vi "PS Control-alternate.vi"() -> ()   [LabVIEW 2020]
panel:
  out "Power Supply State":T1(ring)
  out "Output Cluster":T2 {"MaxLambdaCurrent [A]" format="%.2f"; "LambdaRates [A/min]" format="%.5e"; "MaxNormalCurrent [A]" format="%.2f"; "StabilitySetting [%]" format="%.2f"; "FieldCurrentRatio [T/A]" format="%.2f"; "SwitchWaitTime [s]" format="%.2f"; "SwitchHtrCurrent [mA]" format="%.2f"; "TrainRates [A/min]" format="%.5e"; "NormalRates [A/min]" format="%.5e"; "Breakpts [A]" format="%.5e"}
  in  "Local Enable":bool
  in  "Lambda Mode":bool
  in  "Training Mode":bool
  out "Lambda":bool
  out "Train":bool
  out "Persistent Field":dbl format="%.4f"
  out "Persistence Status":string
  out "Persistent":bool
  in  "Return from persistence":bool
  in  "Make Persistent":bool
  in  "Ramp to Zero":bool
  in  "Hold":bool
  in  "Ramp to Setpoint":bool
  in  "Rate [T/min]":dbl min=0.0 max=5.0 step=0.1 format="%.5f"
  in  "Setpoint [T]":dbl format="%.5f"
  out "Magnet \nVoltage":dbl format="%.2f"
  out "Field [T]":dbl format="%.4f"
  out "Switch Heater Error":bool
  out "Switch heater \nconfirmed":bool
  out "Switch Heater":bool
  in  "VISA session":refnum<visa-resource-name>="GPIB0::22::INSTR"
  in  "stop":bool
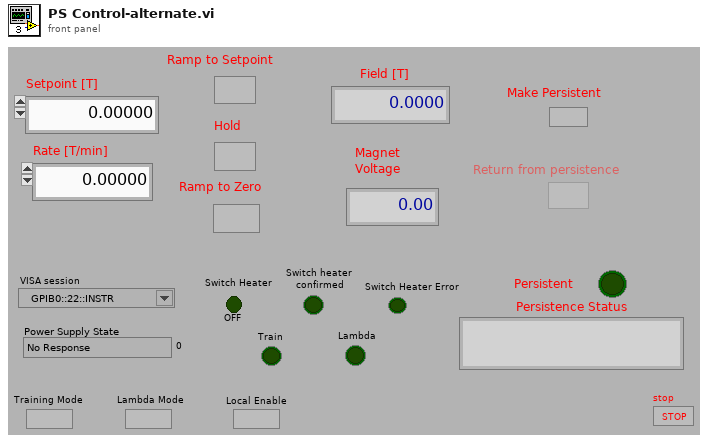
[diagram p1: front panel]
types:
  T1 = enum16{"No Response", "Ramping to programmed field ", "Holding at programmed field", "Paused", "Ramp Manual Up", "Ramp Manual Down", "Ramping to Zero", "QUENCH", "Heating Persistence Switch", "At Zero Current"}
  T2 = cluster{"Breakpts [A]":dbl[], "NormalRates [A/min]":dbl[], "TrainRates [A/min]":dbl[], "SwitchHtrCurrent [mA]":dbl, "SwitchWaitTime [s]":dbl, "FieldCurrentRatio [T/A]":dbl, "StabilitySetting [%]":dbl, "MaxNormalCurrent [A]":dbl, "Magnet ID":string, "LambdaRates [A/min]":dbl[], "MaxLambdaCurrent [A]":dbl}
  T3 = enum16{"Normal", "Train", "Lambda", "Train & Lambda"}
  T4 = enum8{"Enabled", "Disabled", "Disabled and Grayed Out"}
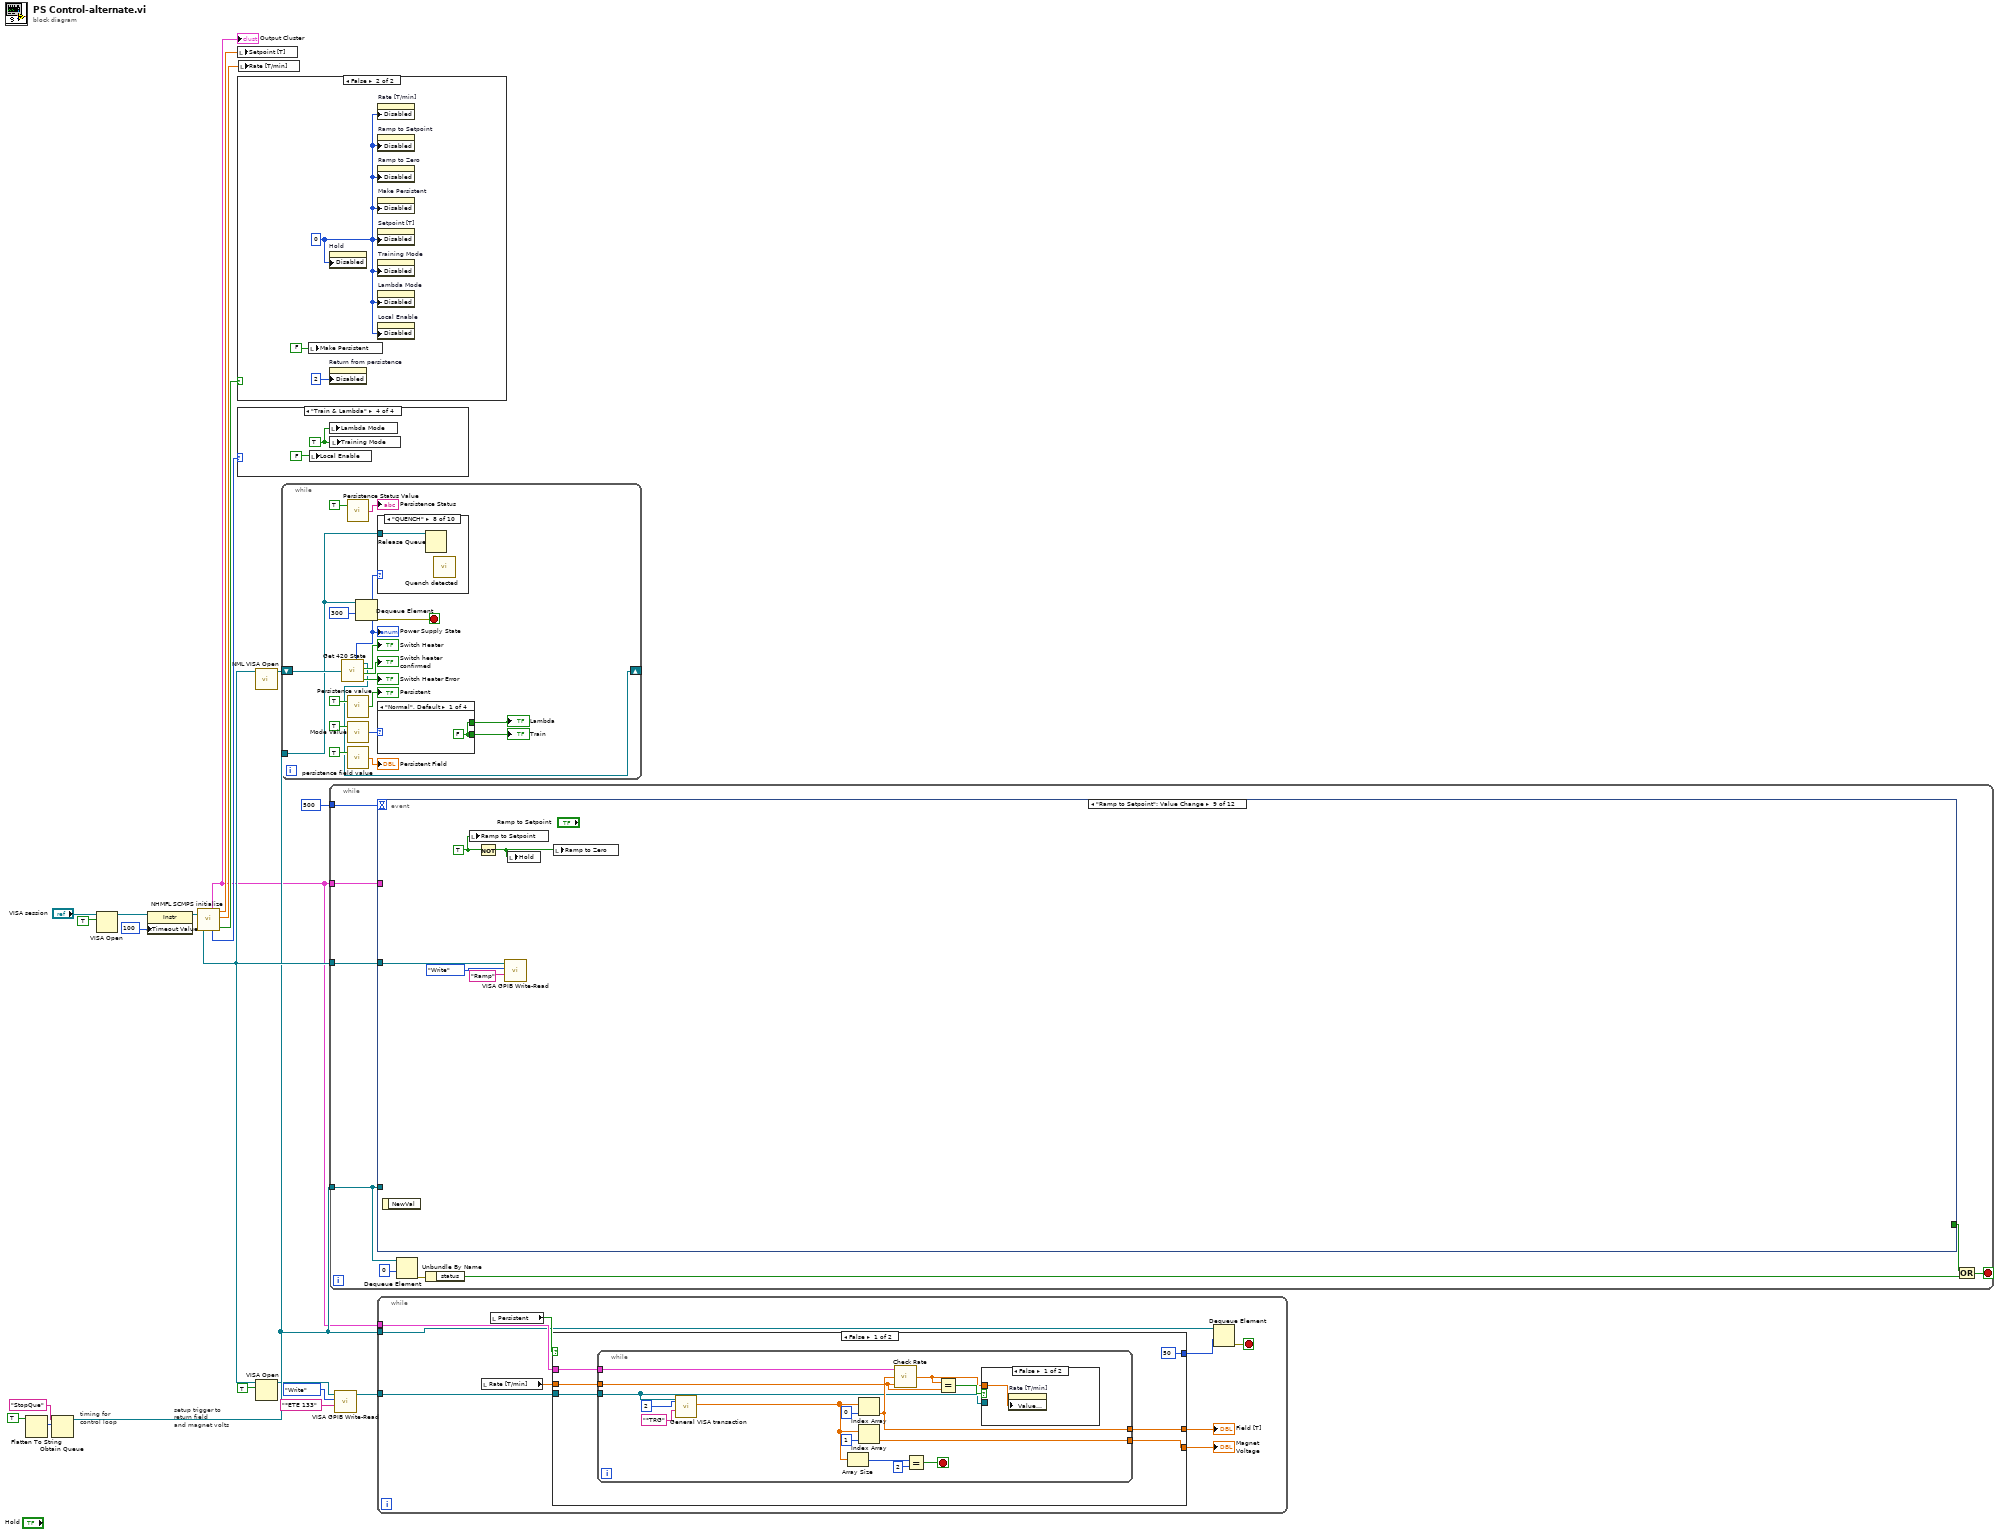
[diagram p0: block diagram]
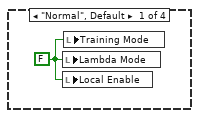
[diagram p2: hidden frame]
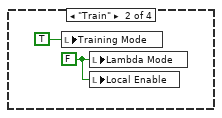
[diagram p3: hidden frame]
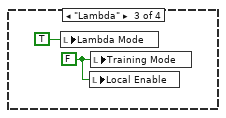
[diagram p4: hidden frame]
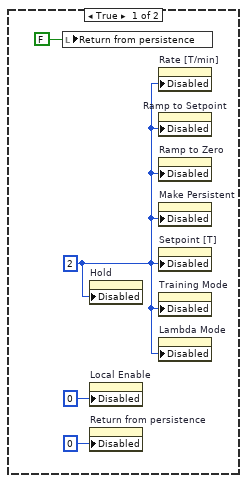
[diagram p5: hidden frame]
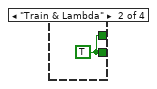
[diagram p15: hidden frame]
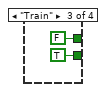
[diagram p16: hidden frame]
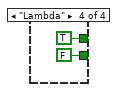
[diagram p17: hidden frame]
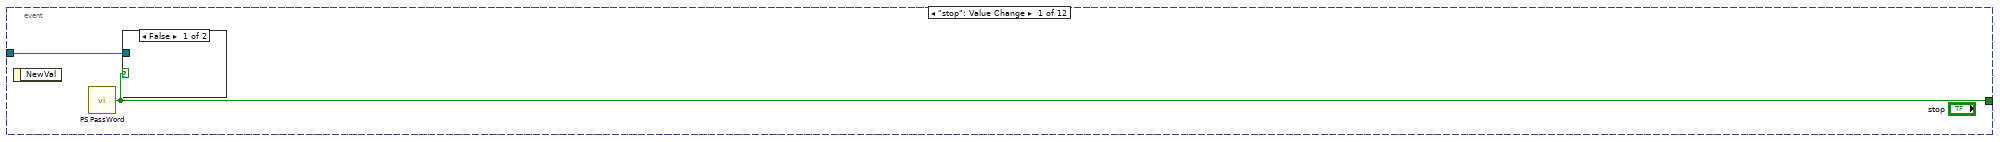
[diagram p18: hidden frame]
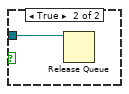
[diagram p19: hidden frame]
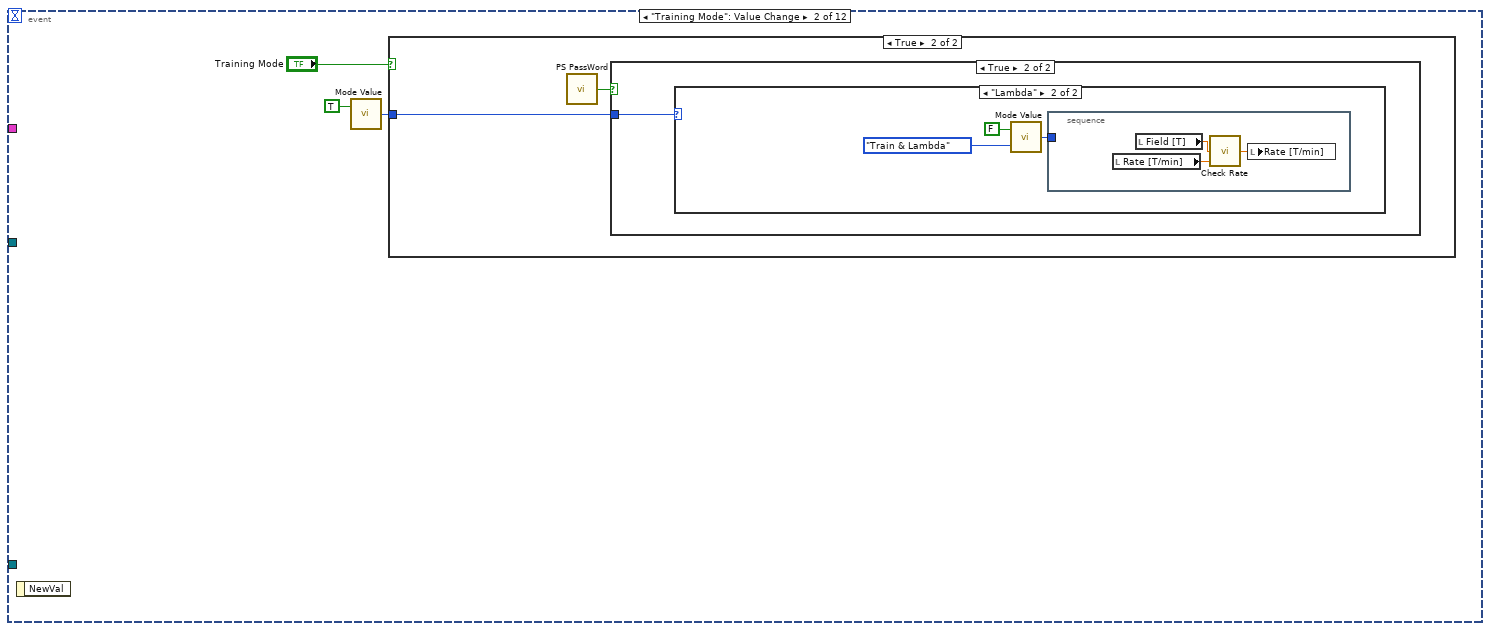
[diagram p20: hidden frame]
diagram:
  # "timing for \ncontrol loop"
  # "setup trigger to \nreturn field\nand magnet volts"
  n1 = Flatten To String(anything=TRUE) -> (type string=w18:i16[])  [unwired: 3 in, 2 out]
  n2 = Obtain Queue(name (unnamed)="StopQue", element data type=w18) -> (queue out=w13:refnum<queue>)  [unwired: 3 in, 2 out]
  n3 = VISA Open(duplicate session (F)=TRUE, VISA resource name="VISA session") -> (VISA resource name=w2:refnum<visa-resource-name>)  [unwired: 3 in, 1 out]
  n4 = property class="Instr"(reference=w2, "General Settings:Timeout Value"=u32 100) -> (reference out=w6:refnum<visa-resource-name>)  [unwired: 1 in, 1 out]
  n5 = call "NHMFL SCMPS initialize.vi"("VISA session"=w6) -> ("dup VISA session"=w14:refnum<visa-resource-name>, "Output Cluster"=w9:T2, "Mode Out"=w11:T3, "Programmed Field"=w16:dbl, "Ramp Rate"=w10:dbl, "Persistent"=w12:bool)  [unwired: 1 out]
  "Output Cluster" <- w9
  n6 = local write "Setpoint [T]"(w16) -> ()
  n7 = case shown="False" w12 {
    frame True {
      w24 = 2
      n8 = local write "Return from persistence"(FALSE ("Return from persistence")) -> ()
      n9 = property on="Hold" class="Bool (strict)"("Disabled"=w24) -> ()  [unwired: 2 in, 2 out]
      n10 = property on="Local Enable" class="Bool (strict)"("Disabled"=u8 0) -> ()  [unwired: 2 in, 2 out]
      n11 = property on="Return from persistence" class="Bool (strict)"("Disabled"=u8 0) -> ()  [unwired: 2 in, 2 out]
      n12 = property on="Rate [T/min]" class="DigNum (strict)"("Disabled"=w24) -> ()  [unwired: 2 in, 2 out]
      n13 = property on="Ramp to Setpoint" class="Bool (strict)"("Disabled"=w24) -> ()  [unwired: 2 in, 2 out]
      n14 = property on="Ramp to Zero" class="Bool (strict)"("Disabled"=w24) -> ()  [unwired: 2 in, 2 out]
      n15 = property on="Make Persistent" class="Bool (strict)"("Disabled"=w24) -> ()  [unwired: 2 in, 2 out]
      n16 = property on="Setpoint [T]" class="DigNum (strict)"("Disabled"=w24) -> ()  [unwired: 2 in, 2 out]
      n17 = property on="Training Mode" class="Bool (strict)"("Disabled"=w24) -> ()  [unwired: 2 in, 2 out]
      n18 = property on="Lambda Mode" class="Bool (strict)"("Disabled"=w24) -> ()  [unwired: 2 in, 2 out]
    }
    frame False {
      w27 = 0
      n19 = local write "Make Persistent"(FALSE ("Return from persistence")) -> ()
      n20 = property on="Hold" class="Bool (strict)"("Disabled"=w27) -> ()  [unwired: 2 in, 2 out]
      n21 = property on="Return from persistence" class="Bool (strict)"("Disabled"=u8 2) -> ()  [unwired: 2 in, 2 out]
      n22 = property on="Rate [T/min]" class="DigNum (strict)"("Disabled"=w27) -> ()  [unwired: 2 in, 2 out]
      n23 = property on="Ramp to Setpoint" class="Bool (strict)"("Disabled"=w27) -> ()  [unwired: 2 in, 2 out]
      n24 = property on="Ramp to Zero" class="Bool (strict)"("Disabled"=w27) -> ()  [unwired: 2 in, 2 out]
      n25 = property on="Make Persistent" class="Bool (strict)"("Disabled"=w27) -> ()  [unwired: 2 in, 2 out]
      n26 = property on="Setpoint [T]" class="DigNum (strict)"("Disabled"=w27) -> ()  [unwired: 2 in, 2 out]
      n27 = property on="Training Mode" class="Bool (strict)"("Disabled"=w27) -> ()  [unwired: 2 in, 2 out]
      n28 = property on="Lambda Mode" class="Bool (strict)"("Disabled"=w27) -> ()  [unwired: 2 in, 2 out]
      n29 = property on="Local Enable" class="Bool (strict)"("Disabled"=w27) -> ()  [unwired: 2 in, 2 out]
    }
  }
  n30 = case shown="\"Train & Lambda\"" w11 {
    frame "Normal", Default {
      w30 = FALSE ("Training Mode")
      n31 = local write "Lambda Mode"(w30) -> ()
      n32 = local write "Local Enable"(w30) -> ()
      n33 = local write "Training Mode"(w30) -> ()
    }
    frame "Train" {
      w32 = FALSE
      n34 = local write "Training Mode"(TRUE) -> ()
      n35 = local write "Lambda Mode"(w32) -> ()
      n36 = local write "Local Enable"(w32) -> ()
    }
    frame "Lambda" {
      w33 = FALSE
      n37 = local write "Lambda Mode"(TRUE) -> ()
      n38 = local write "Local Enable"(w33) -> ()
      n39 = local write "Training Mode"(w33) -> ()
    }
    frame "Train & Lambda" {
      w35 = TRUE
      n40 = local write "Local Enable"(FALSE) -> ()
      n41 = local write "Lambda Mode"(w35) -> ()
      n42 = local write "Training Mode"(w35) -> ()
    }
  }
  n43 = local write "Rate [T/min]"(w10) -> ()
  n44 = call "NML VISA Open.vi"("VISA resource name"=w14) -> ("VISA resource name out"=w3:refnum<visa-resource-name>)  [unwired: 9 in, 1 out]
  n45 = VISA Open(duplicate session (F)=TRUE, VISA resource name=w14) -> (VISA resource name=w5:refnum<visa-resource-name>)  [unwired: 3 in, 1 out]
  n46 = while {
    tunnel: w13 -> [w41]
    shift-right: [w37] -> _
    shift-left: w3 -> [w53]
    stop <- w52 stop-if-true
    n47 = call "Get 420 State.vi"("VISA session"=w53) -> ("State"=w40:T1, "dup VISA session"=w37:refnum<visa-resource-name>, "Switch Heater"=→"Switch Heater":bool, "Switch heater \nconfirmed"=→"Switch heater \nconfirmed":bool, "Switch Heater Error"=→"Switch Heater Error":bool)  [unwired: 1 out]
    "Power Supply State" <- w40
    n48 = call "Persistence Status Value.vi"("Read/Write this vi"=TRUE) -> ("Persistence Status Out"=→"Persistence Status":string)  [unwired: 1 in]
    n49 = call "Persistence value.vi"("Read/Write this vi"=TRUE) -> ("Persistence Out"=→"Persistent":bool)  [unwired: 1 in]
    n50 = call "Mode Value.vi"("Read/Write this vi"=TRUE) -> ("Mode Out"=w45:T3)  [unwired: 1 in]
    n51 = call "persistence field value.vi"("Read/Write this vi"=TRUE) -> ("Persistent Field Out"=→"Persistent Field":dbl)  [unwired: 1 in]
    n52 = Dequeue Element(queue=w41, timeout in ms (-1)=300) -> (error out=w52:errorcluster)  [unwired: 1 in, 3 out]
    n53 = case shown="\"QUENCH\"" w40 {
      tunnel: w41 -> [_ _ _ _ _ _ _ w56 _ _]
      frame "No Response", Default {
      }
      frame "Ramping to programmed field " {
      }
      frame "Holding at programmed field" {
      }
      frame "Paused" {
      }
      frame "Ramp Manual Up" {
      }
      frame "Ramp Manual Down" {
      }
      frame "Ramping to Zero" {
      }
      frame "QUENCH" {
        n54 = Release Queue(queue=w56) -> ()  [unwired: 2 in, 3 out]
        n55 = call "Quench detected.vi"() -> ()  [unwired: 1 out]
      }
      frame "Heating Persistence Switch" {
      }
      frame "At Zero Current" {
      }
    }
    n56 = case shown="\"Normal\", Default" w45 {
      tunnel: [w57 w58 TRUE FALSE] -> w44
      tunnel: [w57 w58 FALSE TRUE] -> w43
      frame "Normal", Default {
        w57 = FALSE
      }
      frame "Train & Lambda" {
        w58 = TRUE
      }
      frame "Train" {
      }
      frame "Lambda" {
      }
    }
    "Train" <- w44
    "Lambda" <- w43
  }
  n57 = while {
    tunnel: w14 -> [w71]
    tunnel: 500 ("y") -> [w70]
    tunnel: w13 -> [w67]
    tunnel: w9 -> [w68]
    stop <- w65 stop-if-true
    n58 = event shown="[8] \"Ramp to Setpoint\": Value Change" {
      selector: _ -> [_ _ _ _ _ _ _ _ _ _ _ _]
      dyn-events: _ -> [_ _ _ _ _ _ _ _ _ _ _ _]
      timeout: w70 -> [_ _ _ _ _ _ _ _ _ _ _ _]
      tunnel: w71 -> [_ _ _ w125 w147 w190 w200 w224 w230 w233 w238 _]
      tunnel: w67 -> [w73 _ _ _ _ _ _ _ _ _ _ _]
      tunnel: [w72 _ _ _ _ _ _ _ _ _ _ _] -> w69
      tunnel: w68 -> [_ _ _ w124 w141 _ _ w221 _ _ _ _]
      event "stop": Value Change {
        n59 = event-data() -> ()  [unwired: 1 in, 1 out]
        n60 = call "PS PassWord.vi"() -> ("Password Correct"=w72:bool)  [unwired: 2 in]
        n61 = case shown="False" w72 {
          tunnel: w73 -> [_ w74]
          frame False {
          }
          frame True {
            n62 = Release Queue(queue=w74) -> ()  [unwired: 2 in, 3 out]
          }
        }
      }
      event "Training Mode": Value Change {
        n63 = event-data() -> ()  [unwired: 1 in, 1 out]
        n64 = call "Mode Value.vi"("Read/Write this vi"=TRUE) -> ("Mode Out"=w75:T3)  [unwired: 1 in]
        n65 = case shown="True" "Training Mode" {
          tunnel: w75 -> [w78 w83]
          frame False {
            n66 = case shown="\"Train\", Default" w78 {
              frame "Train", Default {
                n67 = call "Mode Value.vi"("Mode In"=T3."Normal", "Read/Write this vi"=FALSE) -> ()  [unwired: 1 out]
              }
              frame "Train & Lambda" {
                n68 = call "Mode Value.vi"("Mode In"=T3."Lambda", "Read/Write this vi"=FALSE) -> ()  [unwired: 1 out]
              }
            }
          }
          frame True {
            n69 = call "PS PassWord.vi"() -> ("Password Correct"=w84:bool)  [unwired: 2 in]
            n70 = case shown="True" w84 {
              tunnel: w83 -> [_ w86]
              frame False {
                n71 = local write "Training Mode"(FALSE ("Train")) -> ()
              }
              frame True {
                n72 = case shown="\"Lambda\"" w86 {
                  frame "Normal", Default {
                    n73 = call "Mode Value.vi"("Mode In"=T3."Train", "Read/Write this vi"=FALSE) -> ("Mode Out"=w87:T3)
                    n74 = stacked-sequence {
                      tunnel: w87 -> [_]
                      frame #0 {
                        n75 = local read "Rate [T/min]"() -> (w92:dbl)
                        n76 = local read "Field [T]"() -> (w91:dbl)
                        n77 = call "Check Rate.vi"("Rate"=w92, "Field"=w91) -> ("Checked Rate"=w90:dbl)  [unwired: 1 in]
                        n78 = local write "Rate [T/min]"(w90) -> ()
                      }
                    }
                  }
                  frame "Lambda" {
                    n79 = call "Mode Value.vi"("Mode In"=T3."Train & Lambda", "Read/Write this vi"=FALSE) -> ("Mode Out"=w93:T3)
                    n80 = stacked-sequence {
                      tunnel: w93 -> [_]
                      frame #0 {
                        n81 = local read "Rate [T/min]"() -> (w98:dbl)
                        n82 = local read "Field [T]"() -> (w97:dbl)
                        n83 = call "Check Rate.vi"("Rate"=w98, "Field"=w97) -> ("Checked Rate"=w96:dbl)  [unwired: 1 in]
                        n84 = local write "Rate [T/min]"(w96) -> ()
                      }
                    }
                  }
                }
              }
            }
          }
        }
      }
      event "Lambda Mode": Value Change {
        n85 = event-data() -> ()  [unwired: 1 in, 1 out]
        n86 = call "Mode Value.vi"("Read/Write this vi"=TRUE) -> ("Mode Out"=w99:T3)  [unwired: 1 in]
        n87 = case shown="False" "Lambda Mode" {
          tunnel: w99 -> [w102 w107]
          frame False {
            n88 = case shown="\"Lambda\", Default" w102 {
              frame "Lambda", Default {
                n89 = call "Mode Value.vi"("Mode In"=T3."Normal", "Read/Write this vi"=FALSE) -> ()  [unwired: 1 out]
              }
              frame "Train & Lambda" {
                n90 = call "Mode Value.vi"("Mode In"=T3."Train", "Read/Write this vi"=FALSE) -> ()  [unwired: 1 out]
              }
            }
          }
          frame True {
            n91 = call "PS PassWord.vi"() -> ("Password Correct"=w108:bool)  [unwired: 2 in]
            n92 = case shown="True" w108 {
              tunnel: w107 -> [_ w110]
              frame False {
                n93 = local write "Lambda Mode"(FALSE) -> ()
              }
              frame True {
                n94 = case shown="\"Train\"" w110 {
                  frame "Train" {
                    n95 = call "Mode Value.vi"("Mode In"=T3."Train & Lambda", "Read/Write this vi"=FALSE) -> ("Mode Out"=w111:T3)
                    n96 = stacked-sequence {
                      tunnel: w111 -> [_]
                      frame #0 {
                        n97 = local read "Rate [T/min]"() -> (w116:dbl)
                        n98 = local read "Field [T]"() -> (w115:dbl)
                        n99 = call "Check Rate.vi"("Rate"=w116, "Field"=w115) -> ("Checked Rate"=w114:dbl)  [unwired: 1 in]
                        n100 = local write "Rate [T/min]"(w114) -> ()
                      }
                    }
                  }
                  frame "Normal", Default {
                    n101 = call "Mode Value.vi"("Mode In"=T3."Lambda", "Read/Write this vi"=FALSE) -> ("Mode Out"=w117:T3)
                    n102 = stacked-sequence {
                      tunnel: w117 -> [_]
                      frame #0 {
                        n103 = local read "Rate [T/min]"() -> (w122:dbl)
                        n104 = local read "Field [T]"() -> (w121:dbl)
                        n105 = call "Check Rate.vi"("Rate"=w122, "Field"=w121) -> ("Checked Rate"=w120:dbl)  [unwired: 1 in]
                        n106 = local write "Rate [T/min]"(w120) -> ()
                      }
                    }
                  }
                }
              }
            }
          }
        }
      }
      event "Local Enable": Value Change {
        n107 = event-data() -> ("NewVal"=w123:bool)  [unwired: 1 in]
        n108 = case shown="False" w123 {
          tunnel: w125 -> [w127 w133]
          tunnel: w124 -> [_ w132]
          frame False {
            n109 = call "VISA GPIB Write-Read.vi"("Command"="SYST:REM" ("Command String"), "Action"=enum16{"Write", "Read", "Write & Read"}."Write", "VISA resource name"=w127) -> ("dup VISA Session"=w126:refnum<visa-resource-name>)  [unwired: 5 in, 3 out]
            n110 = stacked-sequence {
              tunnel: w126 -> [_]
              frame #0 {
                n111 = local write "Local Enable"(FALSE ("Local Enable")) -> ()
              }
            }
          }
          frame True {
            n112 = call "PS PassWord.vi"() -> ("Password Correct"=w131:bool)  [unwired: 2 in]
            n113 = case shown="True" w131 {
              tunnel: w133 -> [_ w136]
              tunnel: w132 -> [_ _]
              frame False {
                n114 = local write "Local Enable"(FALSE) -> ()
              }
              frame True {
                n115 = call "VISA GPIB Write-Read.vi"("Command"="SYST:LOC" ("Command String"), "Action"=enum16{"Write", "Read", "Write & Read"}."Write", "VISA resource name"=w136) -> ("dup VISA Session"=w135:refnum<visa-resource-name>)  [unwired: 5 in, 3 out]
                n116 = stacked-sequence {
                  tunnel: w135 -> [_]
                  frame #0 {
                    n117 = local write "Local Enable"(TRUE) -> ()
                  }
                }
              }
            }
          }
        }
      }
      event "Setpoint [T]": Value Change {
        n118 = event-data() -> ()  [unwired: 1 in, 1 out]
        n119 = call "Mode Value.vi"("Read/Write this vi"=TRUE) -> ("Mode Out"=w143:T3)  [unwired: 1 in]
        n120 = case shown="\"Train & Lambda\"" w143 {
          tunnel: "Setpoint [T]" -> [w151 w160 w170 w180]
          tunnel: w141 -> [w158 w168 w178 w188]
          tunnel: [w150 w162 w172 w182] -> w140
          frame "Normal", Default {
            n121 = Unbundle By Name(w158) -> ("MaxNormalCurrent [A]"=w156:dbl, "FieldCurrentRatio [T/A]"=w155:dbl)
            n122 = Multiply(x=w156, y=w155) -> (x*y=w157:dbl)
            n123 = Absolute Value(x=w151) -> (abs(x)=w154:dbl)
            n124 = In Range and Coerce(upper limit=w157, x=w154, lower limit=0.0) -> (coerced(x)=w152:dbl)  [unwired: 1 out]
            n125 = Sign(1:w151) -> (0:w149:dbl)
            n126 = Multiply(x=w152, y=w149) -> (x*y=w150:dbl)
          }
          frame "Train" {
            n127 = Unbundle By Name(w168) -> ("MaxNormalCurrent [A]"=w166:dbl, "FieldCurrentRatio [T/A]"=w165:dbl)
            n128 = Multiply(x=w166, y=w165) -> (x*y=w167:dbl)
            n129 = Absolute Value(x=w160) -> (abs(x)=w164:dbl)
            n130 = In Range and Coerce(upper limit=w167, x=w164, lower limit=0.0) -> (coerced(x)=w161:dbl)  [unwired: 1 out]
            n131 = Sign(1:w160) -> (0:w159:dbl)
            n132 = Multiply(x=w161, y=w159) -> (x*y=w162:dbl)
          }
          frame "Lambda" {
            n133 = Unbundle By Name(w178) -> ("MaxLambdaCurrent [A]"=w176:dbl, "FieldCurrentRatio [T/A]"=w175:dbl)
            n134 = Multiply(x=w176, y=w175) -> (x*y=w177:dbl)
            n135 = Absolute Value(x=w170) -> (abs(x)=w174:dbl)
            n136 = In Range and Coerce(upper limit=w177, x=w174, lower limit=0.0) -> (coerced(x)=w171:dbl)  [unwired: 1 out]
            n137 = Sign(1:w170) -> (0:w169:dbl)
            n138 = Multiply(x=w171, y=w169) -> (x*y=w172:dbl)
          }
          frame "Train & Lambda" {
            n139 = Unbundle By Name(w188) -> ("MaxLambdaCurrent [A]"=w186:dbl, "FieldCurrentRatio [T/A]"=w185:dbl)
            n140 = Multiply(x=w186, y=w185) -> (x*y=w187:dbl)
            n141 = Absolute Value(x=w180) -> (abs(x)=w184:dbl)
            n142 = In Range and Coerce(upper limit=w187, x=w184, lower limit=0.0) -> (coerced(x)=w181:dbl)  [unwired: 1 out]
            n143 = Sign(1:w180) -> (0:w179:dbl)
            n144 = Multiply(x=w181, y=w179) -> (x*y=w182:dbl)
          }
        }
        n145 = local write "Setpoint [T]"(w140) -> ()
        n146 = Format Into String(format string="CONF:FIELD:PROG %f" ("Command String"), w140) -> (resulting string=w146:string)  [unwired: 2 in, 1 out]
        n147 = call "VISA GPIB Write-Read.vi"("Command"=w146, "Action"=enum16{"Write", "Read", "Write & Read"}."Write", "VISA resource name"=w147) -> ()  [unwired: 5 in, 4 out]
      }
      event "Make Persistent": Value Change {
        n148 = event-data() -> ()  [unwired: 1 in, 1 out]
        n149 = flat-sequence {
          tunnel: w190 -> [w191]
          tunnel: [w191] -> w189
          tunnel: w189 -> [w194]
          frame #0 {
            w193 = u8 2 ("Disabled")
            # "Disable Controls"
            n150 = property on="Persistence Status" class="Str"("Blinking"=TRUE) -> ()  [unwired: 2 in, 2 out]
            n151 = property on="Hold" class="Bool (strict)"("Disabled"=w193) -> ()  [unwired: 2 in, 2 out]
            n152 = property on="Training Mode" class="Bool (strict)"("Disabled"=w193) -> ()  [unwired: 2 in, 2 out]
            n153 = property on="Return from persistence" class="Bool (strict)"("Disabled"=w193) -> ()  [unwired: 2 in, 2 out]
            n154 = property on="Rate [T/min]" class="DigNum (strict)"("Disabled"=w193) -> ()  [unwired: 2 in, 2 out]
            n155 = property on="Lambda Mode" class="Bool (strict)"("Disabled"=w193) -> ()  [unwired: 2 in, 2 out]
            n156 = property on="Local Enable" class="Bool (strict)"("Disabled"=w193) -> ()  [unwired: 2 in, 2 out]
            n157 = property on="Ramp to Setpoint" class="Bool (strict)"("Disabled"=w193) -> ()  [unwired: 2 in, 2 out]
            n158 = property on="Ramp to Zero" class="Bool (strict)"("Disabled"=w193) -> ()  [unwired: 2 in, 2 out]
            n159 = property on="Setpoint [T]" class="DigNum (strict)"("Disabled"=w193) -> ()  [unwired: 2 in, 2 out]
            n160 = property on="Make Persistent" class="Bool (strict)"("Disabled"=w193) -> ()  [unwired: 2 in, 2 out]
          }
          frame #1 {
            # "make persistent routine"
            n161 = call "NML SCMPS make persistent.vi"("VISA session"=w194) -> ()  [unwired: 1 in, 3 out]
          }
          frame #2 {
            # "enable return from persistence control"
            n162 = local write "Return from persistence"(FALSE ("Return from persistence")) -> ()
            n163 = property on="Persistence Status" class="Str"("Blinking"=FALSE) -> ()  [unwired: 2 in, 2 out]
            n164 = property on="Return from persistence" class="Bool (strict)"("Disabled"=u8 0) -> ()  [unwired: 2 in, 2 out]
          }
        }
      }
      event "Return from persistence": Value Change {
        n165 = event-data() -> ()  [unwired: 1 in, 1 out]
        n166 = flat-sequence {
          tunnel: w200 -> [w201]
          tunnel: [w201] -> w199
          tunnel: w199 -> [w204]
          tunnel: [w204] -> w198
          tunnel: w198 -> [w205]
          frame #0 {
            w203 = u8 2 ("Disabled")
            # "disable both controls (others should already be disabled)"
            n167 = property on="Persistence Status" class="Str"("Blinking"=TRUE) -> ()  [unwired: 2 in, 2 out]
            n168 = property on="Return from persistence" class="Bool (strict)"("Disabled"=w203) -> ()  [unwired: 2 in, 2 out]
            n169 = property on="Make Persistent" class="Bool (strict)"("Disabled"=w203) -> ()  [unwired: 2 in, 2 out]
          }
          frame #1 {
            # "run return from persistence vi"
            n170 = call "NML SCMPS unpersistence.vi"("VISA session"=w204) -> ()  [unwired: 2 in, 3 out]
          }
          frame #2 {
            # "enable all controls except return from persistence \nand change rate back to normal"
            n171 = local read "Rate [T/min]"() -> (w212:dbl)
            n172 = Format Into String(format string="CONF:RAMP:RATE:FIELD %f" ("Command String"), w212) -> (resulting string=w211:string)  [unwired: 2 in, 1 out]
            n173 = local read "Setpoint [T]"() -> (w207:dbl)
            n174 = call "VISA GPIB Write-Read.vi"("Command"=w211, "Action"=enum16{"Write", "Read", "Write & Read"}."Write", "VISA resource name"=w205) -> ("dup VISA Session"=w206:refnum<visa-resource-name>)  [unwired: 5 in, 3 out]
            n175 = Format Into String(format string="CONF:FIELD:PROG %f" ("Command String"), w207) -> (resulting string=w208:string)  [unwired: 2 in, 1 out]
            n176 = call "VISA GPIB Write-Read.vi"("Command"=w208, "Action"=enum16{"Write", "Read", "Write & Read"}."Write", "VISA resource name"=w206) -> ()  [unwired: 5 in, 4 out]
          }
          frame #3 {
            (unwired) FALSE (".not. x?")
            w216 = T4."Enabled" ("Disabled")
            w215 = FALSE
            # "enable all controls except return from persistence \nand change rate back to normal"
            n177 = local write "Hold"(TRUE) -> ()
            n178 = local write "Make Persistent"(w215) -> ()
            n179 = property on="Persistence Status" class="Str"("Blinking"=w215) -> ()  [unwired: 2 in, 2 out]
            n180 = local write "Ramp to Setpoint"(w215) -> ()
            n181 = local write "Ramp to Zero"(w215) -> ()
            n182 = property on="Hold" class="Bool (strict)"("Disabled"=w216) -> ()  [unwired: 2 in, 2 out]
            n183 = property on="Lambda Mode" class="Bool (strict)"("Disabled"=w216) -> ()  [unwired: 2 in, 2 out]
            n184 = property on="Setpoint [T]" class="DigNum (strict)"("Disabled"=w216) -> ()  [unwired: 2 in, 2 out]
            n185 = property on="Training Mode" class="Bool (strict)"("Disabled"=w216) -> ()  [unwired: 2 in, 2 out]
            n186 = property on="Ramp to Zero" class="Bool (strict)"("Disabled"=w216) -> ()  [unwired: 2 in, 2 out]
            n187 = property on="Local Enable" class="Bool (strict)"("Disabled"=w216) -> ()  [unwired: 2 in, 2 out]
            n188 = property on="Make Persistent" class="Bool (strict)"("Disabled"=w216) -> ()  [unwired: 2 in, 2 out]
            n189 = property on="Rate [T/min]" class="DigNum (strict)"("Disabled"=w216) -> ()  [unwired: 2 in, 2 out]
            n190 = property on="Ramp to Setpoint" class="Bool (strict)"("Disabled"=w216) -> ()  [unwired: 2 in, 2 out]
          }
        }
      }
      event "Rate [T/min]": Value Change {
        n191 = event-data() -> ()  [unwired: 1 in, 1 out]
        n192 = local read "Field [T]"() -> (w220:dbl)
        n193 = call "Check Rate.vi"("Rate"="Rate [T/min]", "Field"=w220, "input cluster"=w221) -> ("Checked Rate"=w218:dbl)
        n194 = local write "Rate [T/min]"(w218) -> ()
        n195 = Format Into String(format string="CONF:RAMP:RATE:FIELD %f" ("Command String"), w218) -> (resulting string=w223:string)  [unwired: 2 in, 1 out]
        n196 = call "VISA GPIB Write-Read.vi"("Command"=w223, "Action"=enum16{"Write", "Read", "Write & Read"}."Write", "VISA resource name"=w224) -> ()  [unwired: 5 in, 4 out]
      }
      event "Ramp to Setpoint": Value Change {
        w226 = TRUE
        n197 = event-data() -> ()  [unwired: 1 in, 1 out]
        n198 = local write "Ramp to Setpoint"(w226) -> ()
        n199 = Not(x=w226) -> (.not. x?=w227:bool)
        n200 = call "VISA GPIB Write-Read.vi"("Command"="Ramp" ("Command String"), "Action"=enum16{"Write", "Read", "Write & Read"}."Write", "VISA resource name"=w230) -> ()  [unwired: 5 in, 4 out]
        n201 = local write "Hold"(w227) -> ()
        n202 = local write "Ramp to Zero"(w227) -> ()
      }
      event "Hold": Value Change {
        w231 = TRUE
        n203 = event-data() -> ()  [unwired: 1 in, 1 out]
        n204 = local write "Hold"(w231) -> ()
        n205 = call "VISA GPIB Write-Read.vi"("Command"="PAUSE" ("Command String"), "Action"=enum16{"Write", "Read", "Write & Read"}."Write", "VISA resource name"=w233) -> ()  [unwired: 5 in, 4 out]
        n206 = Not(x=w231) -> (.not. x?=w232:bool)
        n207 = local write "Ramp to Setpoint"(w232) -> ()
        n208 = local write "Ramp to Zero"(w232) -> ()
      }
      event "Ramp to Zero": Value Change {
        w236 = TRUE
        n209 = event-data() -> ()  [unwired: 1 in, 1 out]
        n210 = local write "Ramp to Zero"(w236) -> ()
        n211 = Not(x=w236) -> (.not. x?=w237:bool)
        n212 = call "VISA GPIB Write-Read.vi"("Command"="ZERO" ("Command String"), "Action"=enum16{"Write", "Read", "Write & Read"}."Write", "VISA resource name"=w238) -> ()  [unwired: 5 in, 4 out]
        n213 = local write "Hold"(w237) -> ()
        n214 = local write "Ramp to Setpoint"(w237) -> ()
      }
      event Timeout {
        n215 = event-data() -> ()  [unwired: 1 in, 1 out]
      }
    }
    n216 = Dequeue Element(queue=w67, timeout in ms (-1)=0) -> (error out=w66:errorcluster)  [unwired: 1 in, 3 out]
    n217 = Unbundle By Name(w66) -> ("status"=w64:bool)
    n218 = Or(x=w69, y=w64) -> (x .or. y?=w65:bool)
  }
  n219 = call "VISA GPIB Write-Read.vi"("Command"="*ETE 133" ("Command String"), "Action"=enum16{"Write", "Read", "Write & Read"}."Write", "VISA resource name"=w5) -> ("dup VISA Session"=w21:refnum<visa-resource-name>)  [unwired: 5 in, 3 out]
  n220 = while {
    tunnel: w21 -> [w249]
    tunnel: w13 -> [w242]
    tunnel: w9 -> [w243]
    stop <- w246 stop-if-true
    n221 = local read "Rate [T/min]"() -> (w241:dbl)
    n222 = local read "Persistent"() -> (w245:bool)
    n223 = case shown="False" w245 {
      tunnel: w249 -> [w255 _]
      tunnel: [w252 w274] -> w248
      tunnel: [w254 0] -> w247
      tunnel: [50 ("Field display timing [ms]") 100] -> w244
      tunnel: w243 -> [w251 _]
      tunnel: w241 -> [w250 _]
      frame False {
        n224 = while {
          tunnel: w255 -> [w256]
          tunnel: [w270] -> w254
          tunnel: [w269] -> w252
          tunnel: w251 -> [w268]
          tunnel: w250 -> [w259]
          stop <- w260 stop-if-true
          n225 = call "General VISA transaction.vi"("Wait (mS)"=u32 2 ("wait (mS)"), "Command String"="*TRG", "VISA Session"=w256) -> ("Measurement"=w263:dbl[])  [unwired: 3 in, 5 out]
          n226 = Array Size(array=w263) -> (size(s)=w262:i32)
          n227 = Index Array(array=w263, index=0) -> (element=w269:dbl)
          n228 = Index Array(array=w263, index=1) -> (element=w270:dbl)
          n229 = call "Check Rate.vi"("Rate"=w259, "Field"=w269, "input cluster"=w268) -> ("Checked Rate"=w257:dbl)
          n230 = Equal?(x=w262, y=2) -> (x = y?=w260:bool)
          n231 = Equal?(x=w257, y=w259) -> (x = y?=w258:bool)
          n232 = case shown="False" w258 {
            tunnel: w257 -> [w271 _]
            tunnel: w256 -> [_ _]
            frame False {
              n233 = property on="Rate [T/min]" class="DigNum (strict)"("Value (Signaling)"=w271) -> ()  [unwired: 2 in, 2 out]
            }
            frame True {
            }
          }
        }
      }
      frame True {
        # "slow down if persistent"
        n234 = local read "Persistent Field"() -> (w274:dbl)
      }
    }
    "Field [T]" <- w248
    "Magnet \nVoltage" <- w247
    n235 = Dequeue Element(queue=w242, timeout in ms (-1)=w244) -> (error out=w246:errorcluster)  [unwired: 1 in, 3 out]
  }
